vi "FTW-Benchmark-PublisherSubscriber.vi"() -> ()   [LabVIEW 2013]
uses:
  Actor/src/Message/Base/FTW-Message.lvclass
  Actor/src/Subscriber/FTW-Subscriber.lvclass
  Actor/src/Publisher/FTW-Publisher.lvclass
  Actor/src/Ether/FTW-Ether.lvclass
panel:
  in  "Wait Time for Workers to Start (ms)":u32=500
  in  "Publishers":i32=8
  in  "Published Message Size":u32=1024
  in  "Publish Period":u32=1
  out "Results":cluster{i32, i32, bool, bool}[](array[cluster])
  in  "Send Timeout":i32=-1
  in  "Send Buffer Depth":i32=-1
  in  "Receive Buffer Depth":i32=-1
  in  "Subscribers":i32=8
  in  "Messages":i32=500
  out "Elapsed Time":dbl format="%.6fsec"
  in  "Connection":string(combo)="lvq://*"
  out "Actual Server Address":string
  out "error out":errorcluster
  # "on slower computers and on the first run, not all pubs may\nbe started by the time the first messages are sent\nincrease this timeout if messages are being lost with lots of\npublishers and lots of subscribers and on slower computers"
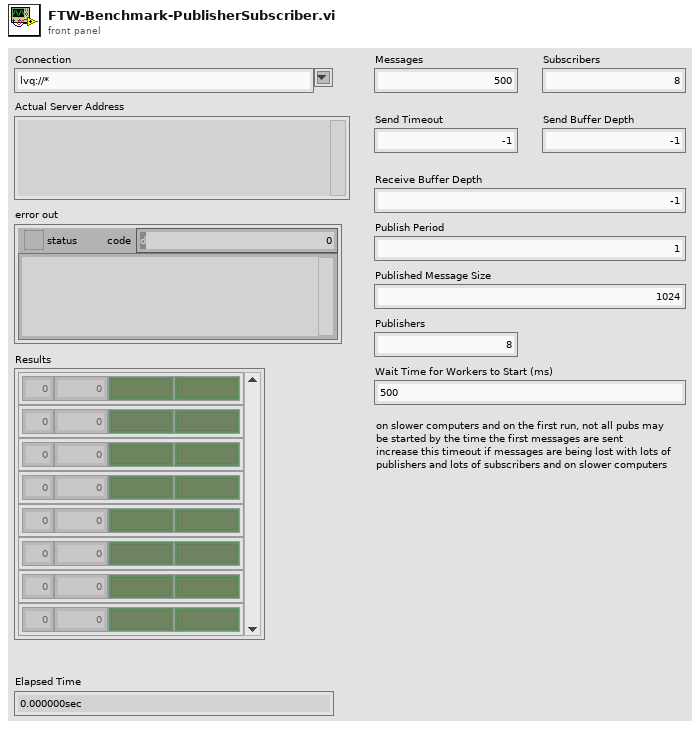
[diagram p1: front panel]
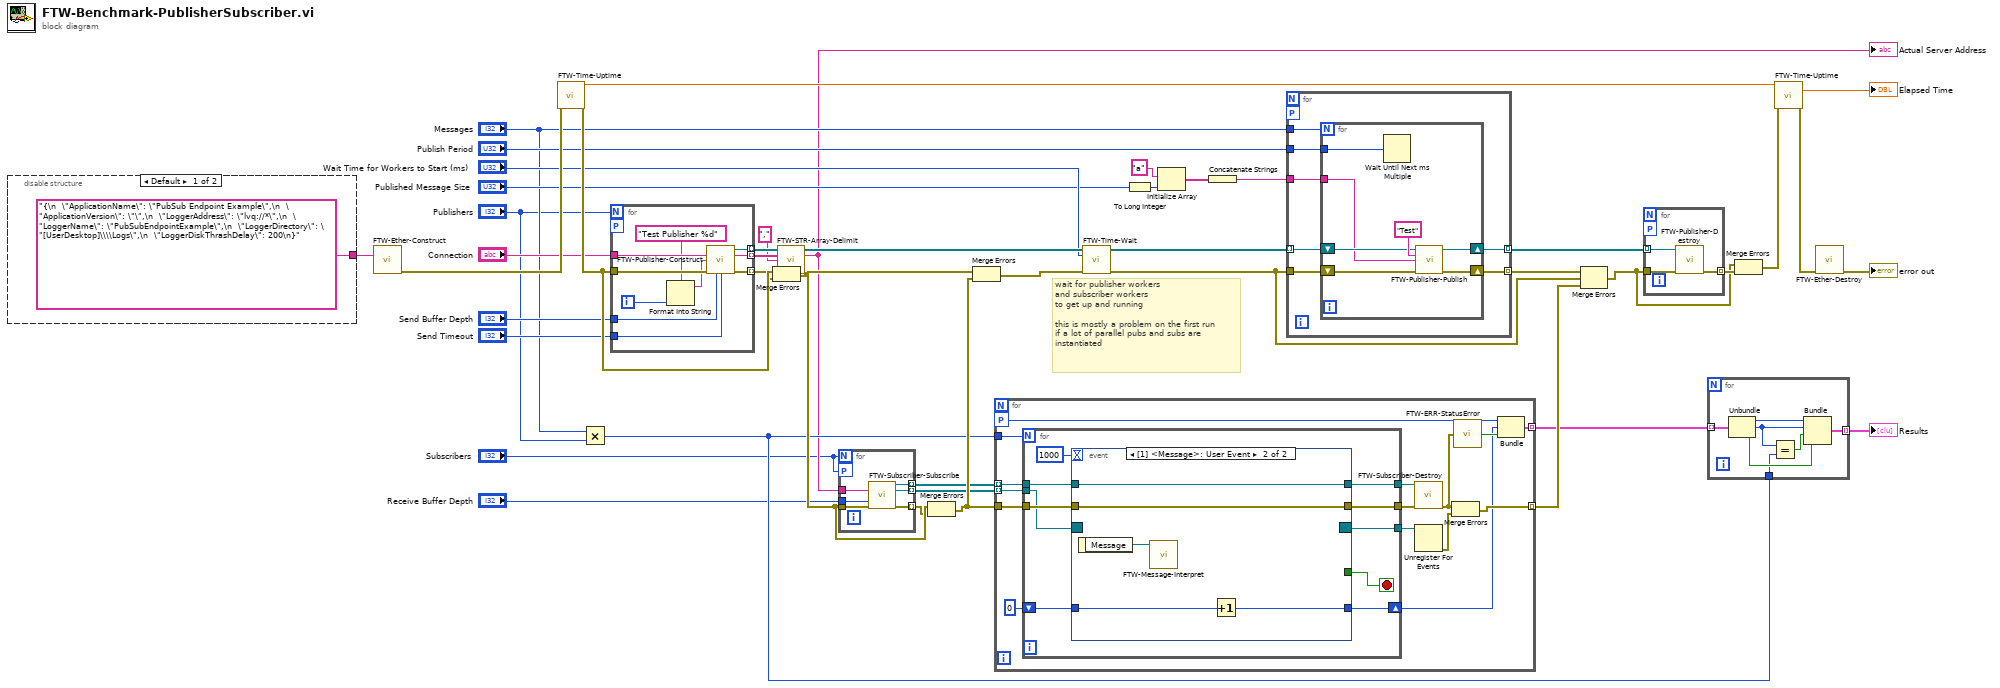
[diagram p0: block diagram]
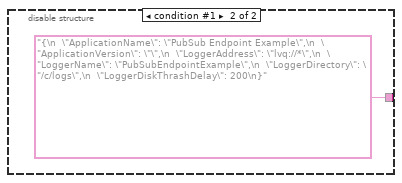
[diagram p2: hidden frame]
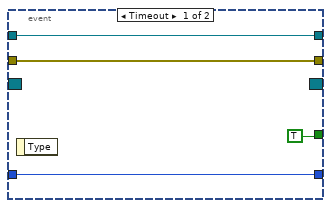
[diagram p3: hidden frame]
diagram:
  # "wait for publisher workers\nand subscriber workers\nto get up and running\n\nthis is mostly a problem on the first run\nif a lot of parallel pubs and subs are\ninstantiated"
  n1 = disable-structure shown="Default" {
    disable-tunnel: ["{\n  \"ApplicationName\": \"PubSub Endpoint Example\",\n  \"ApplicationVersion\": \"\",\n  \"LoggerAddress\": \"lvq://*\",\n  \"LoggerName\": \"PubSubEndpointExample\",\n  \"LoggerDirectory\": \"[UserDesktop]\\\\Logs\",\n  \"LoggerDiskThrashDelay\": 200\n}" ("FTW Ether Configuration") "{\n  \"ApplicationName\": \"PubSub Endpoint Example\",\n  \"ApplicationVersion\": \"\",\n  \"LoggerAddress\": \"lvq://*\",\n  \"LoggerName\": \"PubSubEndpointExample\",\n  \"LoggerDirectory\": \"/c/logs\",\n  \"LoggerDiskThrashDelay\": 200\n}" ("FTW Ether Configuration")] -> w7
    frame condition #0 (active) {
    }
    frame condition #1 {
    }
  }
  n2 = call "FTW-Ether-Construct.vi"("FTW Ether Configuration"=w7) -> ("error out"=w42:errorcluster)  [unwired: 14 in]
  n3 = call "FTW-Time-Uptime.vi"("error in"=w42) -> ("Current Uptime"=w27:dbl, "error out"=w40:errorcluster)  [unwired: 12 in, 1 out]
  n4 = Multiply(x="Messages", y="Publishers") -> (x*y=w8:i32)
  n5 = for {
    N: "Publishers" -> [_]
    tunnel: [w54] -> w34 mode=indexing
    tunnel: [w53] -> w33 mode=indexing
    tunnel: "Connection" -> [w52]
    tunnel: w40 -> [w51]
    tunnel: [w50] -> w25 mode=indexing
    tunnel: "Send Buffer Depth" -> [w49]
    tunnel: "Send Timeout" -> [w48]
    workers-P: _ -> [_]
    i -> [w45]
    n6 = Format Into String(format string="Test Publisher %d" ("Identity"), w45) -> (resulting string=w47:string)  [unwired: 2 in, 1 out]
    n7 = call "FTW-Publisher-Construct.vi"("Address"=w52, "Identity"=w47, "error in"=w51, "Send Buffer Depth (1)"=w49, "Send Timeout (-1)"=w48) -> ("FTW-Publisher Out"=w54:refnum<class "FTW-Publisher.lvclass">, "Actual Address"=w53:string, "error out"=w50:errorcluster)  [unwired: 8 in]
  }
  n8 = Merge Errors(w40, w25) -> (w39:errorcluster)
  n9 = call "FTW-STR-Array-Delimit.vi"("Array of Strings"=w33, "Delimiter"=",") -> ("Delimited String"=w4:string)  [unwired: 13 in]
  "Actual Server Address" <- w4
  n10 = for {
    N: "Subscribers" -> [_]
    tunnel: w39 -> [w60]
    tunnel: [w59] -> w6 mode=indexing
    tunnel: "Receive Buffer Depth" -> [w58]
    tunnel: w4 -> [w57]
    workers-P: "Subscribers" -> [_]
    tunnel: [w56] -> w2 mode=indexing
    tunnel: [w55] -> w1 mode=indexing
    n11 = call "FTW-Subscriber-Subscribe.vi"("Addresses"=w57, "Buffer Depth (1 element)"=w58, "error in"=w60) -> ("FTW-Subscription Out"=w56:refnum<class "FTW-Subscriber.lvclass">, "Subscriber Registration"=w55:refnum<event-registration>, "error out"=w59:errorcluster)  [unwired: 10 in]
  }
  n12 = Merge Errors(w39, w6) -> (w37:errorcluster)
  n13 = Merge Errors(w39, w37) -> (w38:errorcluster)
  n14 = for {
    tunnel: w37 -> [w75]
    tunnel: [w71] -> w22 mode=indexing
    workers-P: _ -> [w69]
    tunnel: [w66] -> w21 mode=indexing
    tunnel: w8 -> [w63]
    tunnel: w2 -> [w62] mode=indexing
    tunnel: w1 -> [w61] mode=indexing
    n15 = for {
      N: w63 -> [_]
      tunnel: w61 -> [w84]
      tunnel: w62 -> [w83]
      tunnel: w75 -> [w85]
      tunnel: [w82] -> w74
      tunnel: [w81] -> w73
      tunnel: [w79] -> w72
      shift-right: [w76] -> w64
      shift-left: 0 -> [w77]
      stop <- w78 stop-if-true
      n16 = event shown="[1] <Message>: User Event" {
        selector: w84 -> [_ _]
        dyn-events: [_ _] -> w79
        timeout: 1000 -> [_ _]
        tunnel: w83 -> [w89 w93]
        tunnel: w85 -> [w88 w92]
        tunnel: [w89 w93] -> w82
        tunnel: [w88 w92] -> w81
        tunnel: [TRUE _] -> w78
        tunnel: [w86 w90] -> w76
        tunnel: w77 -> [w86 w91]
        event Timeout {
          n17 = event-data() -> ()  [unwired: 1 in, 1 out]
        }
        event User Event {
          n18 = event-data() -> ("Message"=w94:refnum<class "FTW-Message.lvclass">)  [unwired: 1 in]
          n19 = call-dynamic "FTW-Message-Interpret.vi"("FTW Message"=w94) -> ()  [unwired: 10 in, 5 out]
          n20 = Increment(x=w91) -> (x+1=w90:i32)
        }
      }
    }
    n21 = call "FTW-Subscriber-Destroy.vi"("FTW-Subscription In"=w74, "error in"=w73) -> ("error out"=w68:errorcluster)  [unwired: 13 in]
    n22 = Unregister For Events(event registration refnum=w72) -> (error out=w70:errorcluster)  [unwired: 1 in]
    n23 = Merge Errors(w68, w70) -> (w71:errorcluster)
    n24 = call "FTW-ERR-StatusError.vi"("error to check"=w68) -> ("Error?"=w67:bool)
    n25 = Bundle(w69, w64, "Error?"=w67) -> (w66:cluster{i32, i32, "Error?":bool})  [unwired: 1 in]
  }
  n26 = call "FTW-Time-Wait.vi"("Wait Time (ms)"="Wait Time for Workers to Start (ms)", "error in"=w38) -> ("error out"=w41:errorcluster)  [unwired: 13 in]
  n27 = To Long Integer(number="Published Message Size") -> (32bit integer=w17:i32)
  n28 = Initialize Array("a", w17) -> (w15:string[])
  n29 = Concatenate Strings(w15) -> (w14:string)
  n30 = for {
    tunnel: [w101] -> w35 mode=indexing
    tunnel: w34 -> [w100] mode=indexing
    tunnel: [w99] -> w31 mode=indexing
    tunnel: w41 -> [w98]
    tunnel: "Messages" -> [w97]
    tunnel: "Publish Period" -> [w96]
    tunnel: w14 -> [w95]
    workers-P: _ -> [_]
    n31 = for {
      N: w97 -> [_]
      tunnel: w96 -> [w103]
      shift-right: [w105] -> w99
      shift-left: w100 -> [w106]
      shift-right: [w107] -> w101
      shift-left: w98 -> [w104]
      tunnel: w95 -> [w102]
      n32 = Wait Until Next ms Multiple(millisecond multiple=w103) -> ()  [unwired: 1 out]
      n33 = call "FTW-Publisher-Publish.vi"("FTW-Publisher In"=w106, "Header"="Test" ("Message Header"), "Body"=w102, "error in"=w104) -> ("FTW-Publisher Out"=w105:refnum<class "FTW-Publisher.lvclass">, "error out"=w107:errorcluster)  [unwired: 10 in]
    }
  }
  n34 = Merge Errors(w35, w41, w22) -> (w11:errorcluster)
  n35 = for {
    tunnel: w11 -> [w111]
    tunnel: [w110] -> w32 mode=indexing
    tunnel: w31 -> [w109] mode=indexing
    workers-P: _ -> [_]
    n36 = call "FTW-Publisher-Destroy.vi"("FTW-Publisher In"=w109, "error in"=w111) -> ("error out"=w110:errorcluster)  [unwired: 13 in]
  }
  n37 = for {
    tunnel: w21 -> [w118] mode=indexing
    tunnel: [w116] -> w20 mode=indexing
    tunnel: w8 -> [w112]
    n38 = Unbundle(w118) -> (w117:i32, w113:i32, "Error?"=w114:bool)
    n39 = Equal?(x=w113, y=w112) -> (x = y?=w115:bool)
    n40 = Bundle(w117, w113, w115, "Error?"=w114) -> (w116:cluster{i32, i32, bool, "Error?":bool})  [unwired: 1 in]
  }
  "Results" <- w20
  n41 = Merge Errors(w11, w32) -> (w12:errorcluster)
  n42 = call "FTW-Time-Uptime.vi"("Previous Uptime"=w27, "error in"=w12) -> ("Elapsed Time"=→"Elapsed Time":dbl, "error out"=w28:errorcluster)  [unwired: 11 in, 1 out]
  n43 = call "FTW-Ether-Destroy.vi"("error in"=w28) -> ("error out"=→"error out":errorcluster)  [unwired: 14 in]
